vi "GlobalAutonVariables.vi"() -> ()   [LabVIEW 2020]
panel:
  out "BR Desired":string[](array[string])
  out "BR Throttle":string[](array[string])
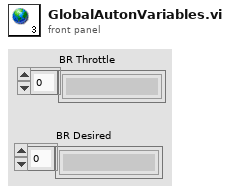
[diagram p1: front panel]
diagram:
